vi "FL_Preprocess_and_save_incrementally_TDMS.vi"(0 "Temporary file output path":path, 1 "Loop iteration":i32, 2 "Offsets, swaps and rotations":T2, 3 "Loop speed in ms":u16, 4 "Save every N seconds":u32=15, 5 "error in (no error)":errorcluster, 6 "Filter type":u16(ring)=5 items=["None", "Kalman 0.50", "Kalman 0.30", "Kalman 0.12", "Savitzky-Golay 3/5", "Savitzky-Golay 3/11", "Savitzky-Golay 3/31"], 7 "Sensor read input":T5(array[cluster]), 8 "Input cluster of SG coefficients":T1, 9 "tdms file in":refnum<k34>, 10 "Pixels per mm":dbl, 11 "Data flow controls in":T4, 12 "Diagram at recording bounds":T3, 13 "Sensor board size":string="Small") -> (14 "Eff. save interval":sgl, 15 "Latest sensor output (decoded)":string[][](array[string]), 16 "Fire TTL":bool, 17 "TTL out N":u8, 18 "Current TTL status":u8, 19 "error out":errorcluster)   [LabVIEW 2018, in "Tracker.lvlib"]
uses:
  Tracker.lvlib
  Controls/CTL_Data_flow_control_cluster.ctl
  <vilib>/Utility/miscctls.llb/LVBoundsTypeDef.ctl
  SW_Globals.vi
  <vilib>/Utility/file.llb/Write Delimited Spreadsheet (string).vi
panel:
  out "Bytes return count":u32
  out "VISA error out":errorcluster
  out "Output to the external terminal":string
  in  "Max chunk size":i64=100000
  in  "Number of the file chunk":u32
  out "Chunk size (in bytes)":i64
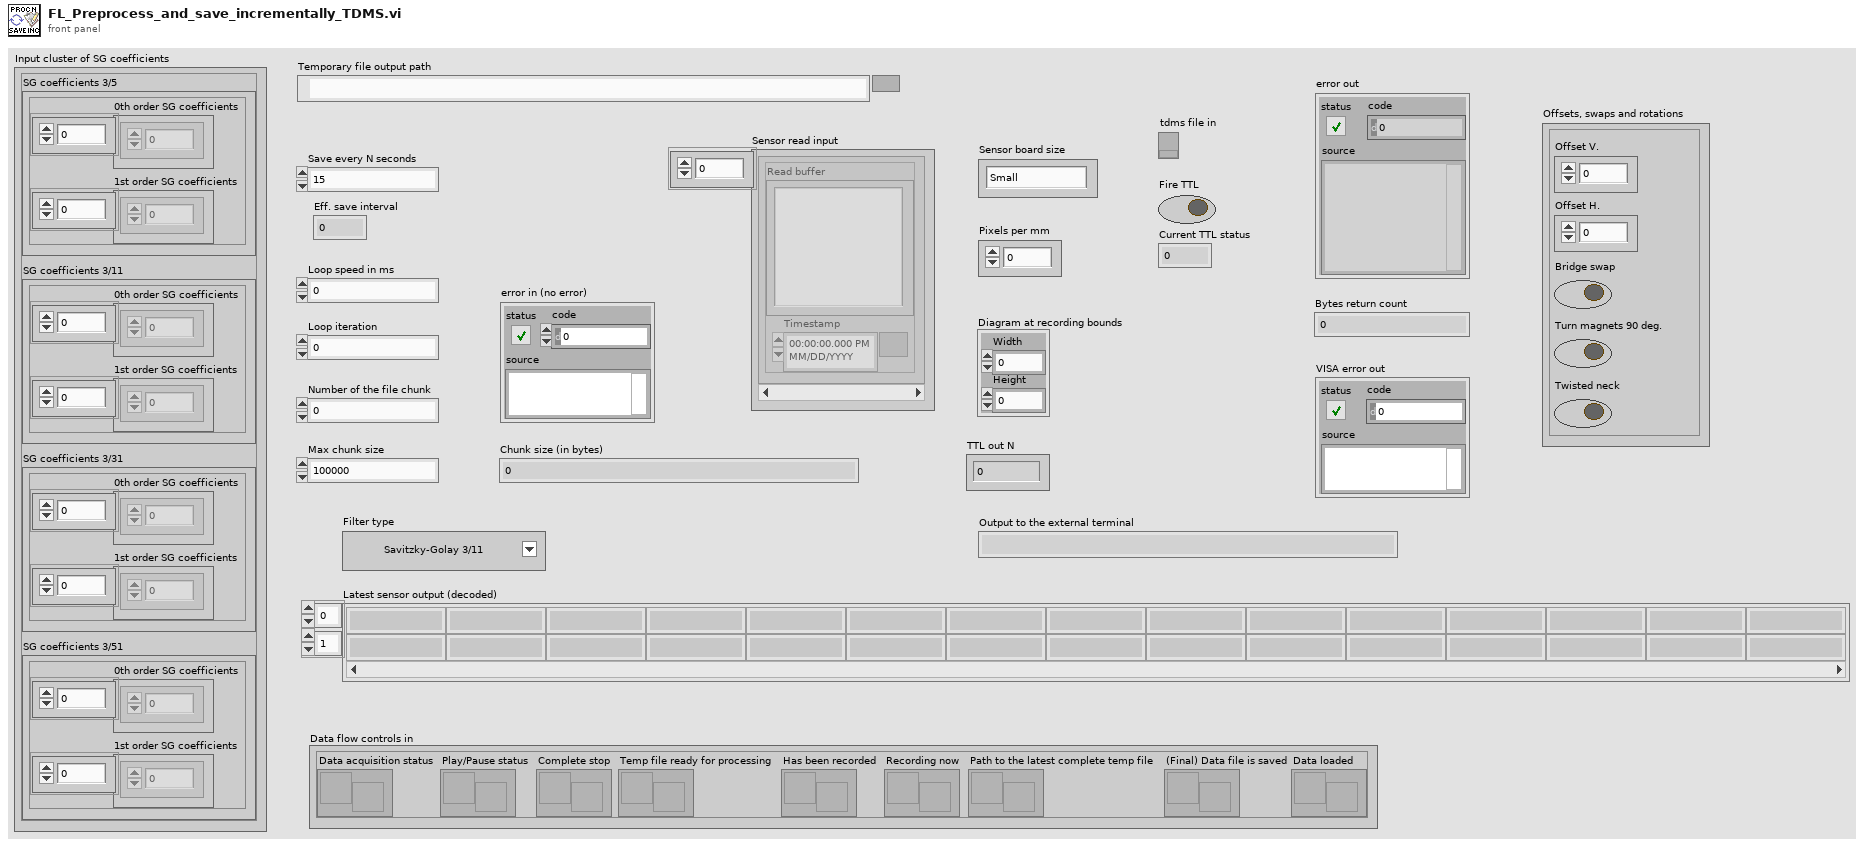
[diagram p1: front panel]
types:
  T1 = cluster{"SG coefficients 3/5":cluster{"0th order SG coefficients":dbl[], "1st order SG coefficients":dbl[]}, "SG coefficients 3/11":cluster{"0th order SG coefficients":dbl[], "1st order SG coefficients":dbl[]}, "SG coefficients 3/31":cluster{"0th order SG coefficients":dbl[], "1st order SG coefficients":dbl[]}, "SG coefficients 3/51":cluster{"0th order SG coefficients":dbl[], "1st order SG coefficients":dbl[]}}
  T2 = cluster{"Offset V.":sgl, "Offset H.":sgl, "Bridge swap":bool, "Turn magnets 90 deg.":bool, "Twisted neck":bool}
  T3 = typedef "LVBoundsTypeDef.ctl" = cluster{"Width":u32, "Height":u32}
  T4 = typedef "Tracker.lvlib/CTL_Data_flow_control_cluster.ctl" = cluster{"Data acquisition status":refnum<notifier>, "Play/Pause status":refnum<notifier>, "Complete stop":refnum<notifier>, "Temp file ready for processing":refnum<notifier>, "Has been recorded":refnum<notifier>, "Recording now":refnum<notifier>, "Path to the latest complete temp file":refnum<notifier>, "(Final) Data file is saved":refnum<notifier>, "Data loaded":refnum<notifier>}
  T5 = cluster{"Read buffer":string, "Timestamp":timestamp}[]
  T6 = cluster{"ms since ON":u32, "delta time":u32, "X1":sgl, "Y1":sgl, "X2":sgl, "Y2":sgl, "TTL inputs":u8, "TTL outputs":u8, "Frame timestamp":timestamp, "Frame OK":bool}
  T7 = cluster{"0th order SG coefficients":dbl[], "1st order SG coefficients":dbl[]}
  T8 = cluster{"X1 filtered":dbl, "Y1 filtered":dbl, "X2 filtered":dbl, "Y2 filtered":dbl, "X1 raw":dbl, "Y1 raw":dbl, "X2 raw":dbl, "Y2 raw":dbl}
  T9 = cluster{"R from center":dbl, "sin(a)":dbl, "Mouse Xc":dbl, "Mouse Yc":dbl, "X1-X2":dbl, "Y1-Y2":dbl, "Cage Xc":dbl, "Cage Yc":dbl}
  T10 = cluster{"R from center":dbl, "phi (mouse angular position in the cage)":dbl, "alpha (mouse rot. angle)":sgl, "X":dbl, "Y":dbl, "theta (from center towards mouse)":dbl, "beta (cage rot. against mouse)":sgl, "w (mouse angle to wall)":dbl}
  T11 = cluster{"Zone[1]":bool, "Zone[2]":bool, "Zone[3]":bool, "Zone[4]":bool, "Zone[5]":bool, "Zone[6]":bool, "Zone[7]":bool, "Zone[8]":bool, "Zone[9]":bool, "Zone[10]":bool, "Zone[11]":bool, "Zone[12]":bool, "Zone[13]":bool}
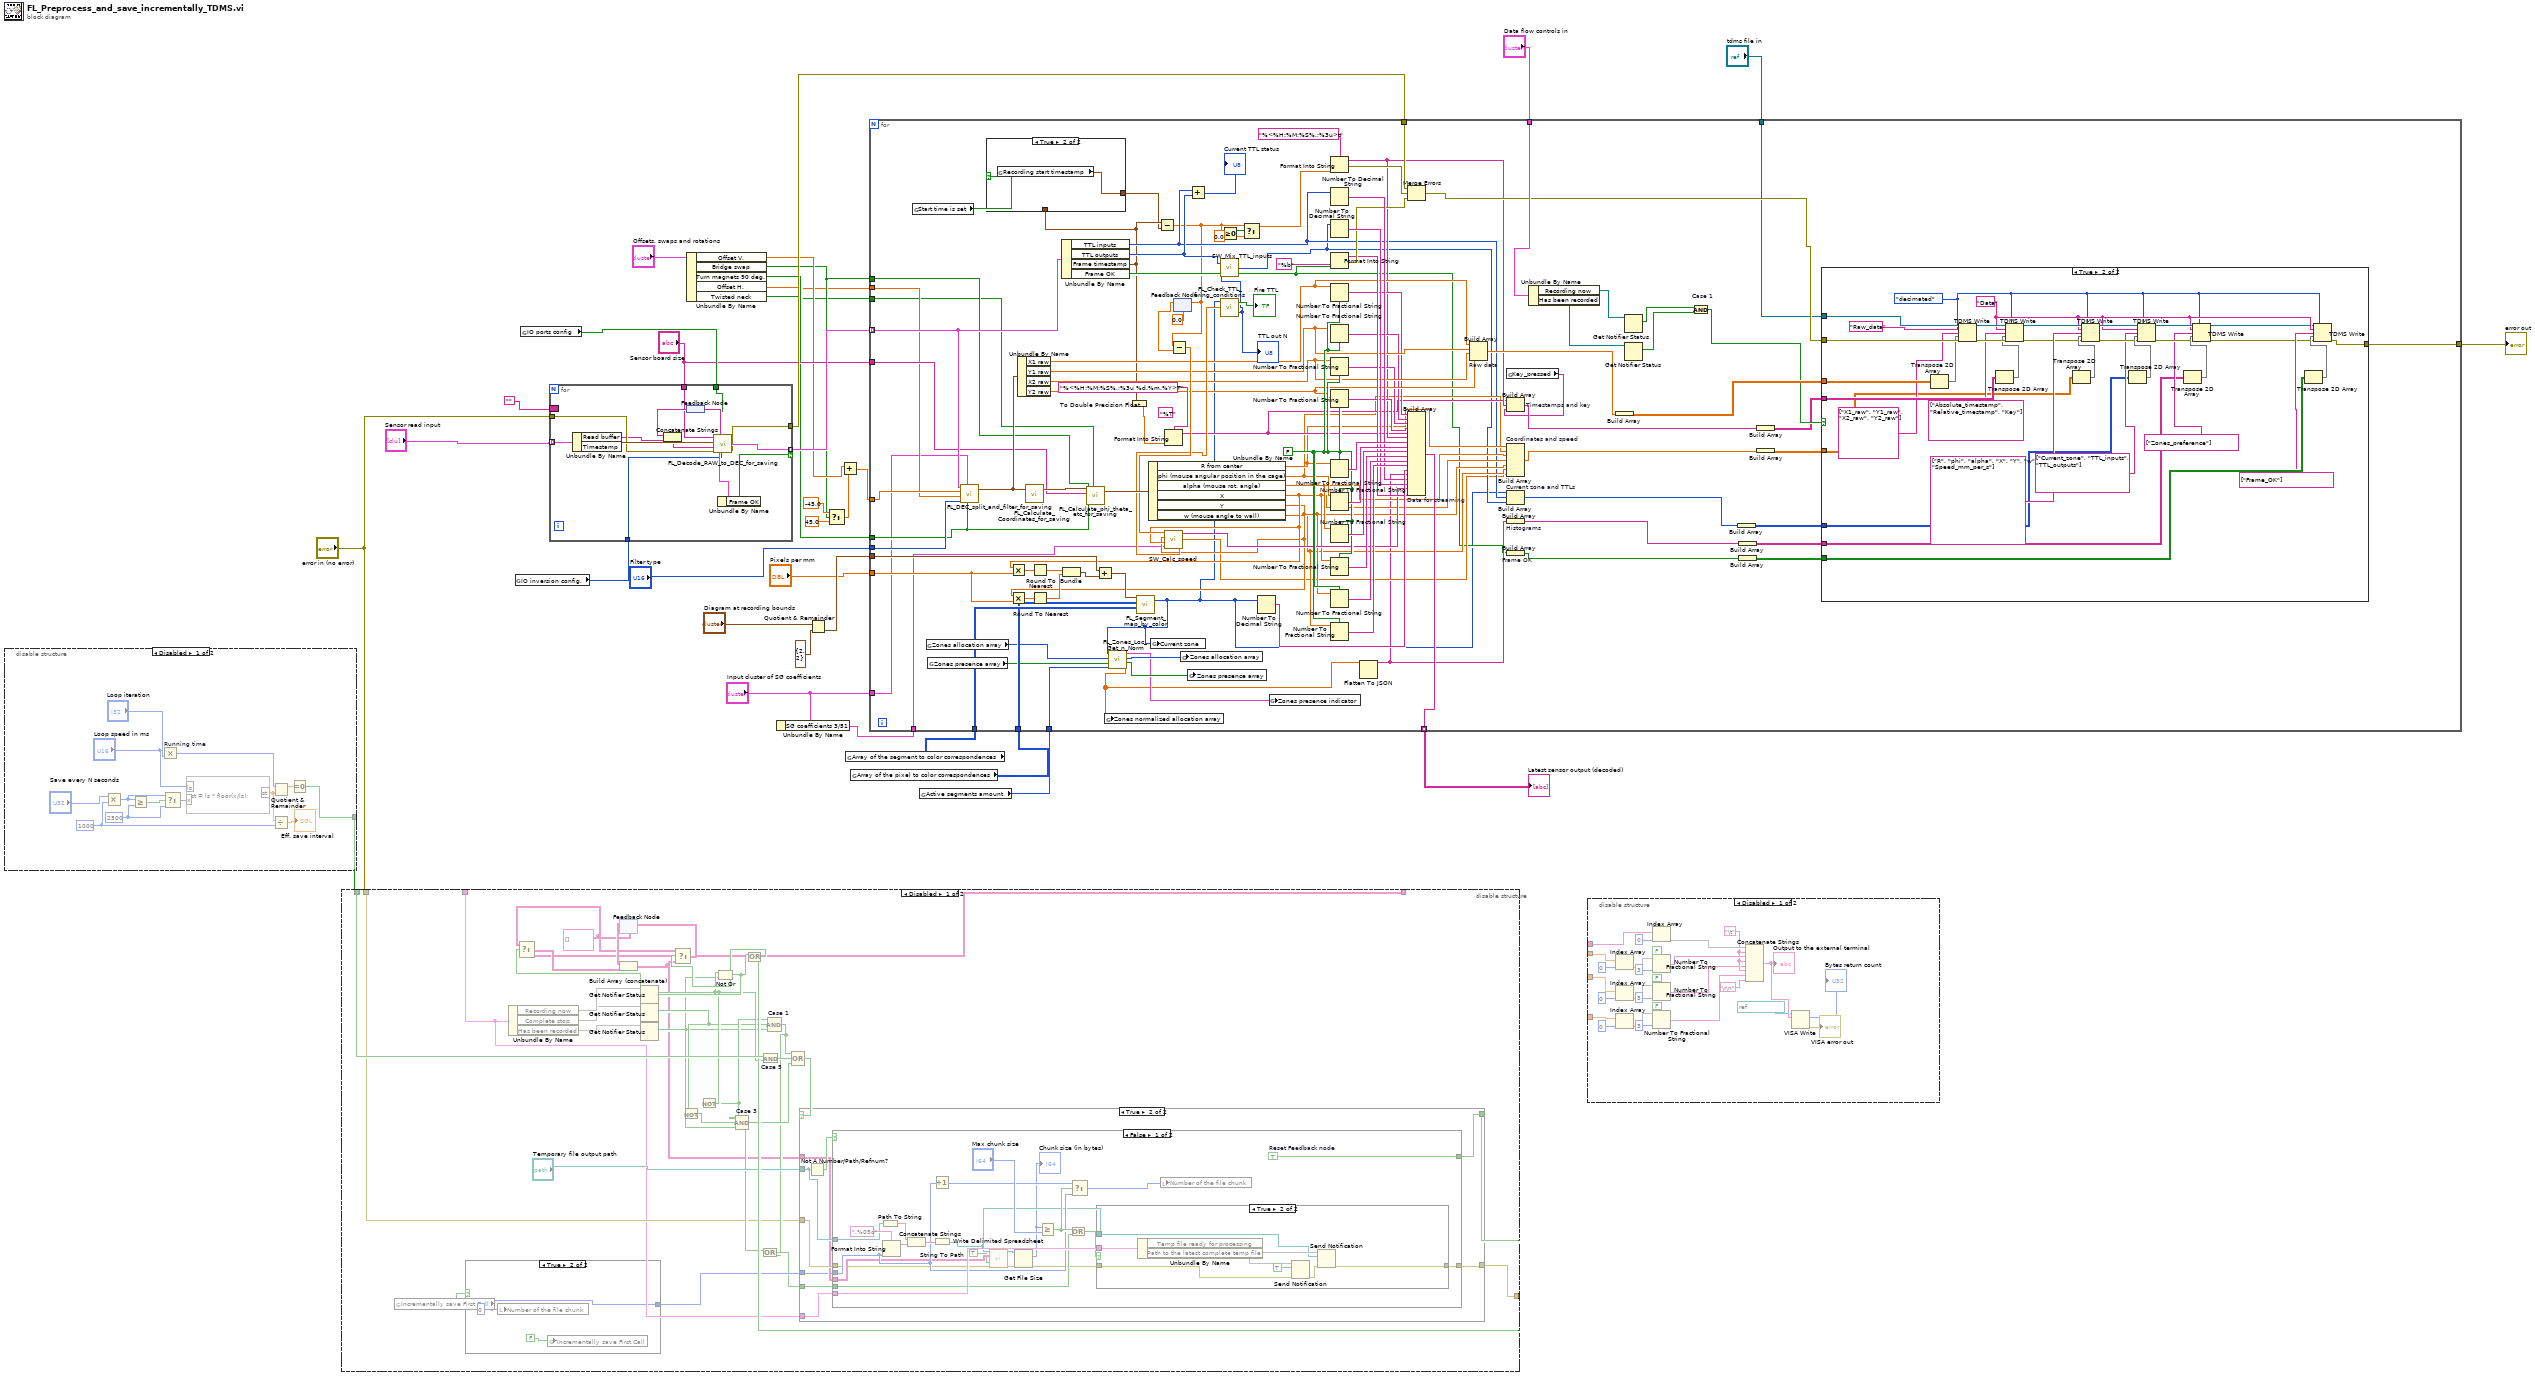
[diagram p0: block diagram]
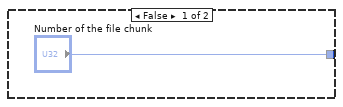
[diagram p2: hidden frame]
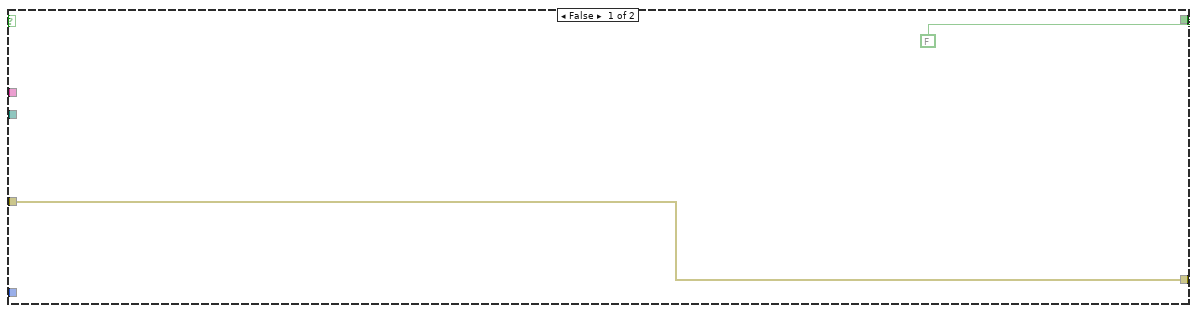
[diagram p3: hidden frame]
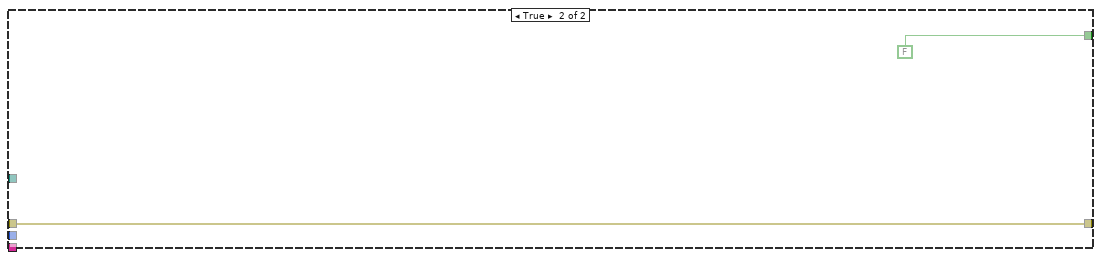
[diagram p5: hidden frame]
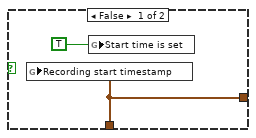
[diagram p9: hidden frame]
diagram:
  n1 = disable-structure shown="Disabled" {
    disable-tunnel: [w44 _] -> w33
    frame Disabled {
      w34 = u32 1000 ("y")
      w41 = 2500
      n2 = Multiply(x="Save every N seconds", y=w34) -> (x*y=w37:u32)
      n3 = Greater Or Equal?(x=w37, y=w41) -> (x >= y?=w42:bool)
      n4 = Multiply "Running time"(x="Loop speed in ms", y="Loop iteration") -> (x*y=w45:i32)
      n5 = Select(t=w37, s=w42, f=w41) -> (s? t:f=w39:u32)
      n6 = formula code="st = ls * floor(x/ls);"("ls"="Loop speed in ms", "x"=w39) -> ("st"=w36:dbl)
      n7 = Divide(x=w36, y=w34) -> (x/y=→"Eff. save interval":dbl)
      n8 = Quotient & Remainder(x=w45, y=w36) -> (x-y*floor(x/y)=w43:dbl)  [unwired: 1 out]
      n9 = Equal To 0?(x=w43) -> (x = 0?=w44:bool)
    }
    frame Enabled {
    }
  }
  n10 = disable-structure shown="Disabled" {
    disable-tunnel: w33 -> [w74 _]
    disable-tunnel: "error in (no error)" -> [w51 _]
    disable-tunnel: [w50 _] -> _
    disable-tunnel: _ -> [w48 _]
    disable-tunnel: _ -> [w47 _]
    frame Disabled {
      w62 = string[][] []
      n11 = global read "SW_Globals.vi" "Incrementally save First Call"() -> (w49:bool)
      n12 = case shown="True" w49 {
        tunnel: ["Number of the file chunk" w78] -> w65
        frame False {
        }
        frame True {
          w78 = 0 ("Number of the file chunk")
          n13 = local write "Number of the file chunk"(w78) -> ()
          n14 = global write "SW_Globals.vi" "Incrementally save First Call"(FALSE ("Incrementally save First Call")) -> ()
        }
      }
      n15 = Unbundle By Name(w47) -> ("Recording now"=w69, "Complete stop"=w68, "Has been recorded"=w67)
      n16 = feedback #1(w62) -> (w72:string[][])
      n17 = Get Notifier Status(notifier=w69) -> (current notification=w59:bool)  [unwired: 1 in, 4 out]
      n18 = Get Notifier Status(notifier=w68) -> (current notification=w57:bool)  [unwired: 1 in, 4 out]
      n19 = Get Notifier Status(notifier=w67) -> (current notification=w56:bool)  [unwired: 1 in, 4 out]
      n20 = Not(x=w57) -> (.not. x?=w55:bool)
      n21 = Not(x=w59) -> (.not. x?=w58:bool)
      n22 = Not Or(1:w56, 2:w59) -> (0:w61:bool)
      n23 = Select(t=w62, s=w61, f=w48) -> (s? t:f=w63:string[][])
      n24 = Build Array (concatenate)(w72, w63) -> (w52:string[][])
      n25 = Compound Arithmetic op=AND "Case 3"(w58, w55, w56) -> (w64:bool)
      n26 = And "Case 5"(x=w74, y=w59) -> (x .and. y?=w75:bool)
      n27 = Compound Arithmetic op=AND "Case 1"(w58, w57, w56) -> (w53:bool)
      n28 = Or(x=w64, y=w53) -> (x .or. y?=w54:bool)
      n29 = Compound Arithmetic op=OR(w53, w75, w64) -> (w73:bool)
      n30 = case shown="True" w73 {
        tunnel: "Temporary file output path" -> [_ w88]
        tunnel: [FALSE w87] -> w70
        tunnel: w51 -> [w79 w86]
        tunnel: [w79 w85] -> w50
        tunnel: w52 -> [_ w84]
        tunnel: w47 -> [_ w83]
        tunnel: w65 -> [_ w82]
        tunnel: w54 -> [_ w81]
        frame False {
        }
        frame True {
          n31 = Not A Number/Path/Refnum?(number/path/refnum=w88) -> (NaN/Path/Refnum?=w89:bool)
          n32 = case shown="False" w89 {
            tunnel: w88 -> [w104 _]
            tunnel: [w95 FALSE] -> w87
            tunnel: w86 -> [w91 w122]
            tunnel: [w102 w122] -> w85
            tunnel: w84 -> [w97 _]
            tunnel: w82 -> [w99 _]
            tunnel: w83 -> [w109 _]
            tunnel: w81 -> [w100 _]
            frame False {
              w95 = TRUE  # Reset Feedback node
              n33 = Path To String(path=w104) -> (string=w106:string)
              n34 = Format Into String(format string=".%05d", w99) -> (resulting string=w107:string)  [unwired: 2 in, 1 out]
              n35 = Concatenate Strings(w106, w107) -> (w108:string)
              n36 = Increment(x=w99) -> (x+1=w111:u32)
              n37 = String To Path(string=w108) -> (path=w98:path)
              n38 = call-poly <vilib>:"Write Delimited Spreadsheet.vi"("file path (dialog if empty)"=w98, "2D data"=w97, "append to file? (new file:F)"=TRUE, "error in (no error)"=w91) -> ("new file path (Not A Path if cancelled)"=w94:path, "error out"=w93:errorcluster)  [unwired: 10 in]
              n39 = Get File Size(file=w94, error in=w93) -> (size (in bytes)=w90:i64, 0:w92:errorcluster)  [unwired: 1 out]
              "Chunk size (in bytes)" <- w90
              n40 = Greater Or Equal?(x=w90, y="Max chunk size") -> (x >= y?=w103:bool)
              n41 = Or(x=w103, y=w100) -> (x .or. y?=w101:bool)
              n42 = Select(t=w111, s=w103, f=w99) -> (s? t:f=w110:u32)
              n43 = case shown="True" w101 {
                tunnel: w109 -> [_ w121]
                tunnel: w98 -> [_ w115]
                tunnel: w92 -> [w113 w117]
                tunnel: [w113 w116] -> w102
                frame False {
                }
                frame True {
                  n44 = Unbundle By Name(w121) -> ("Temp file ready for processing"=w120, "Path to the latest complete temp file"=w119)
                  n45 = Send Notification(notification=TRUE, notifier=w120, error in (no error)=w117) -> (error out=w118:errorcluster)  [unwired: 1 out]
                  n46 = Send Notification(notification=w115, notifier=w119, error in (no error)=w118) -> (error out=w116:errorcluster)  [unwired: 1 out]
                }
              }
              n47 = local write "Number of the file chunk"(w110) -> ()
            }
            frame True {
            }
          }
        }
      }
      n48 = Or(x=w61, y=w70) -> (x .or. y?=w60:bool)
      n49 = Select(t=w62, s=w60, f=w52) -> (s? t:f=w71:string[][])
      n50 = feedback-in #1(w71) -> ()
    }
    frame Enabled {
    }
  }
  n51 = global read "SW_Globals.vi" "IO inversion config."() -> (w16:u16)
  n52 = global read "SW_Globals.vi" "IO ports config"() -> (w18:bool[])
  n53 = for {
    tunnel: "Sensor read input" -> [w136] mode=indexing
    border: "" -> [_]
    tunnel: [w131] -> w30 mode=indexing if=w130
    tunnel: [w129] -> w31
    tunnel: "error in (no error)" -> [w128]
    tunnel: "Sensor board size" -> [w127]
    tunnel: w18 -> [w126]
    tunnel: w16 -> [w124]
    n54 = Unbundle By Name(w136) -> ("Read buffer"=w125:string, "Timestamp"=w135:timestamp)
    n55 = feedback #2() -> (w132:string)
    n56 = Concatenate Strings(w132, w125) -> (w134:string)
    n57 = call "FL_Decode_RAW_to_DEC_for_saving.vi"("Sensor board size"=w127, "IO ports config"=w126, "Input timestamp"=w135, "Input string"=w134, "IO inversion config."=w124, "Error In"=w128) -> ("Output string leftover"=w133:string, "DEC output cluster"=w131:T6, "Error Out"=w129:errorcluster)
    n58 = feedback-in #2(w133) -> ()
    n59 = Unbundle By Name(w131) -> ("Frame OK"=w130:bool)
  }
  n60 = Unbundle By Name("Offsets, swaps and rotations") -> ("Offset V."=w7:sgl, "Bridge swap"=w6:bool, "Turn magnets 90 deg."=w5:bool, "Offset H."=w4:sgl, "Twisted neck"=w3:bool)
  n61 = Unbundle By Name("Input cluster of SG coefficients") -> ("SG coefficients 3/51"=w1:T7)
  n62 = Quotient & Remainder(x="Diagram at recording bounds", y=T3 {"Width"=2, "Height"=2}) -> (floor(x/y)=w25:T3)  [unwired: 1 out]
  n63 = Select(t=sgl -45.0 ("x"), s=w6, f=sgl 45.0 ("x")) -> (s? t:f=w9:sgl)
  n64 = Add(x=w7, y=w9) -> (x+y=w19:sgl)
  n65 = global read "SW_Globals.vi" "Array of the segment to color correspondences"() -> (w23:u32[][])
  n66 = global read "SW_Globals.vi" "Array of the pixel to color correspondences"() -> (w22:u32[][])
  n67 = global read "SW_Globals.vi" "Active segments amount"() -> (w20:u8)
  n68 = for {
    tunnel: w30 -> [w243] mode=indexing
    tunnel: w31 -> [w231]
    tunnel: "Filter type" -> [w230]
    tunnel: w25 -> [w223]
    tunnel: "Pixels per mm" -> [w229]
    tunnel: w23 -> [w221]
    tunnel: w22 -> [w220]
    tunnel: w20 -> [w217]
    tunnel: w19 -> [w144]
    tunnel: w5 -> [w142]
    tunnel: "Sensor board size" -> [w199]
    tunnel: [w176] -> w15 mode=indexing
    tunnel: "tdms file in" -> [w188]
    tunnel: "Data flow controls in" -> [w191]
    tunnel: [w186] -> w12
    tunnel: w6 -> [w145]
    tunnel: w4 -> [w143]
    tunnel: w3 -> [w141]
    tunnel: "Input cluster of SG coefficients" -> [w140]
    tunnel: w1 -> [w139]
    w233 = FALSE ("use system decimal point (T)")
    (unwired) "%T" ("format string")
    n69 = global read "SW_Globals.vi" "Start time is set"() -> (w148:bool)
    n70 = global read "SW_Globals.vi" "Zones allocation array"() -> (w218:i32[])
    n71 = global read "SW_Globals.vi" "Zones presence array"() -> (w216:bool[])
    n72 = call "FL_DEC_split_and_filter_for_saving.vi"("Alternative magnets orientation"=w142, "Input cluster of SG coefficients"=w140, "Filter type"=w230, "Offset H."=w143, "Offset V."=w144, "DEC input cluster"=w243) -> ("Magnets coords"=w245:T8)  [unwired: 1 in]
    n73 = Unbundle By Name(w245) -> ("X1 raw"=w185:dbl, "Y1 raw"=w184:dbl, "X2 raw"=w183:dbl, "Y2 raw"=w182:dbl)
    n74 = call "FL_Calculate_Coordinates_for_saving.vi"("Magnets coords in"=w245) -> ("Output cluster of data"=w244:T9)  [unwired: 2 in]
    n75 = Unbundle By Name(w243) -> ("TTL inputs"=w167:u8, "TTL outputs"=w197:u8, "Frame timestamp"=w147:timestamp, "Frame OK"=w163:bool)
    n76 = case shown="True" w148 {
      tunnel: w147 -> [w246 _]
      tunnel: [w246 w248] -> w146
      frame False {
        n77 = global write "SW_Globals.vi" "Recording start timestamp"(w246) -> ()
        n78 = global write "SW_Globals.vi" "Start time is set"(TRUE ("Start time is set")) -> ()
      }
      frame True {
        n79 = global read "SW_Globals.vi" "Recording start timestamp"() -> (w248:timestamp)
      }
    }
    n80 = call "FL_Calculate_phi_theta_etc_for_saving.vi"("Input cluster of data"=w244, "Sensor board size"=w199, "Bridge swap"=w145, "Use alternative magnets orientation"=w142, "Clamp swap"=w141) -> ("Output data cluster"=w240:T10)  [unwired: 1 in]
    n81 = To Double Precision Float(number=w147) -> (double precision float=w201:dbl)
    n82 = Unbundle By Name(w240) -> ("R from center"=w173:dbl, "phi (mouse angular position in the cage)"=w172:dbl, "alpha (mouse rot. angle)"=w171:sgl, "X"=w170:dbl, "Y"=w169:dbl, "w (mouse angle to wall)"=w168:dbl)
    n83 = Multiply(x=w170, y=w229) -> (x*y=w228:dbl)
    n84 = Multiply(x=w169, y=w229) -> (x*y=w227:dbl)
    n85 = Round To Nearest(number=w228) -> (nearest integer value=w226:dbl)
    n86 = Round To Nearest(number=w227) -> (nearest integer value=w225:dbl)
    n87 = Bundle(w226, w225) -> (w224:cluster{dbl, dbl})  [unwired: 1 in]
    n88 = Add(x=w223, y=w224) -> (x+y=w222:cluster{dbl, dbl})
    n89 = call "FL_Segment_map_by_color.vi"("Array of the segment to color correspondences"=w221, "Array of the pixel to color correspondences"=w220, "Mouse abs. coordinates, pix"=w222) -> ("Current segment' number"=w138:u32)  [unwired: 1 in, 1 out]
    n90 = call "FL_Zones_Loc_Get_n_Norm.vi"("Amount of active segments"=w217, "Zones presence array in"=w216, "Zones allocation array in"=w218, "Current segment' number"=w138) -> ("Zones normalized allocation array out"=w210:dbl[], "Zones presence array out"=w214:bool[], "Zones allocation array out"=w215:i32[], "Zones presence indicator cluster out"=w213:T11)  [unwired: 4 in]
    n91 = global write "SW_Globals.vi" "Zones normalized allocation array"(w210) -> ()
    n92 = global write "SW_Globals.vi" "Current zone"(w138) -> ()
    n93 = Subtract(x=w147, y=w146) -> (x-y=w150:dbl)
    n94 = Format Into String(format string="%<%H:%M:%S%,;%3u %d.%m.%Y>T", w201) -> (resulting string=w174:string)  [unwired: 2 in, 1 out]
    n95 = feedback-in #3(w150) -> ()
    n96 = feedback #3(0.0) -> (w205:dbl)
    n97 = Subtract(x=w150, y=w205) -> (x-y=w203:dbl)
    n98 = call "SW_Calc_speed.vi"("SG coefficients"=w139, "X coord, mm"=w170, "Y coord, mm"=w169, "Time per frame, s"=w203) -> ("Mouse speed for TTL detection, mm/s"=w198:dbl, "Mouse speed, mm/s"=w165:dbl, "Mouse speed for saving, mm/s"=w202:string)
    n99 = global write "SW_Globals.vi" "Zones allocation array"(w215) -> ()
    n100 = global write "SW_Globals.vi" "Zones presence array"(w214) -> ()
    n101 = Add(x=w167, y=w197) -> (x+y=→"Current TTL status":u8)
    n102 = call "FL_Check_TTL_firing_conditions.vi"("Current speed, mm/s"=w198, "Current segment' number (last value)"=w138) -> ("TTL out N"=w196:u8, "Fire TTL"=→"Fire TTL":bool)  [unwired: 1 in]
    "TTL out N" <- w196
    n103 = call "SW_Mix_TTL_inputs.vi"("TTL input 2"=w196, "TTL input 1"=w197) -> ("TTL mixed output"=w166:u8)
    n104 = Greater Or Equal To 0?(x=w150) -> (x >= 0?=w151:bool)
    n105 = Select(t=w150, s=w151, f=0.0) -> (s? t:f=w152:dbl)
    n106 = Number To Decimal String(number=w138) -> (decimal integer string=w219:string)  [unwired: 1 in]
    n107 = global write "SW_Globals.vi" "Zones presence indicator"(w213) -> ()
    n108 = Format Into String(format string="%<%H:%M:%S%.;%3u>t", w152) -> (resulting string=w175:string, error out=w232:errorcluster)  [unwired: 2 in]
    n109 = Number To Decimal String(number=w167) -> (decimal integer string=w211:string)  [unwired: 1 in]
    n110 = Number To Decimal String(number=w166) -> (decimal integer string=w212:string)  [unwired: 1 in]
    n111 = Format Into String(format string="%b", w163) -> (resulting string=w204:string, error out=w209:errorcluster)  [unwired: 2 in]
    n112 = Number To Fractional String(use system decimal point (T)=w233, number=w185) -> (F-format string=w177:string)  [unwired: 2 in]
    n113 = Number To Fractional String(use system decimal point (T)=w233, number=w184) -> (F-format string=w178:string)  [unwired: 2 in]
    n114 = Number To Fractional String(use system decimal point (T)=w233, number=w183) -> (F-format string=w179:string)  [unwired: 2 in]
    n115 = Number To Fractional String(use system decimal point (T)=w233, number=w182) -> (F-format string=w180:string)  [unwired: 2 in]
    n116 = Number To Fractional String(use system decimal point (T)=w233, number=w173) -> (F-format string=w239:string)  [unwired: 2 in]
    n117 = Number To Fractional String(use system decimal point (T)=w233, number=w172) -> (F-format string=w238:string)  [unwired: 2 in]
    n118 = Number To Fractional String(use system decimal point (T)=w233, number=w171) -> (F-format string=w237:string)  [unwired: 2 in]
    n119 = Number To Fractional String(use system decimal point (T)=w233, number=w170) -> (F-format string=w236:string)  [unwired: 2 in]
    n120 = Number To Fractional String(use system decimal point (T)=w233, number=w169) -> (F-format string=w235:string)  [unwired: 2 in]
    n121 = Number To Fractional String(use system decimal point (T)=w233, number=w168) -> (F-format string=w234:string)  [unwired: 2 in]
    n122 = Flatten To JSON(anything=w210) -> (JSON string=w164:string)  [unwired: 2 in, 1 out]
    n123 = Merge Errors(w231, w232, w209) -> (w190:errorcluster)
    n124 = Build Array "Data for streaming"(w177, w178, w179, w180, w174, w175, w239, w238, w237, w236, w235, w234, w219, w164, w211, w212, w202, w204) -> (w176:string[])
    n125 = Build Array "Raw data"(w185, w184, w183, w182) -> (w181:dbl[])
    n126 = global read "SW_Globals.vi" "Key_pressed"() -> (w137:string)
    n127 = Build Array "Timestamps and key"(w174, w175, w137) -> (w162:string[])
    n128 = Build Array "Coordinates and speed"(w173, w172, w171, w170, w169, w168, w165) -> (w160:dbl[])
    n129 = Build Array "Current zone and TTLs"(w138, w167, w166) -> (w158:u32[])
    n130 = Build Array "Histograms"(w164) -> (w156:string[])
    n131 = Build Array "Frame OK"(w163) -> (w154:bool[])
    n132 = Unbundle By Name(w191) -> ("Recording now"=w192:refnum<notifier>, "Has been recorded"=w193:refnum<notifier>)
    n133 = Build Array(w181) -> (w189:dbl[][])
    n134 = Get Notifier Status(notifier=w192) -> (current notification=w194:bool)  [unwired: 1 in, 4 out]
    n135 = Get Notifier Status(notifier=w193) -> (current notification=w195:bool)  [unwired: 1 in, 4 out]
    n136 = And "Case 1"(x=w194, y=w195) -> (x .and. y?=w187:bool)
    n137 = Build Array(w158) -> (w157:u32[][])
    n138 = Build Array(w156) -> (w155:string[][])
    n139 = Build Array(w154) -> (w153:bool[][])
    n140 = Build Array(w162) -> (w161:string[][])
    n141 = Build Array(w160) -> (w159:dbl[][])
    n142 = case shown="True" w187 {
      tunnel: w190 -> [w249 w283]
      tunnel: [w249 w254] -> w186
      tunnel: w189 -> [_ w282]
      tunnel: w161 -> [_ w281]
      tunnel: w188 -> [_ w280]
      tunnel: w159 -> [_ w270]
      tunnel: w157 -> [_ w263]
      tunnel: w155 -> [_ w258]
      tunnel: w153 -> [_ w256]
      frame False {
      }
      frame True {
        w253 = "Data" ("group name in (Untitled)")
        w252 = enum16{"decimated", "interleaved"}."decimated" ("data layout (0:decimated)")
        n143 = Transpose 2D Array(2D array=w282) -> (transposed array=w278:dbl[][])
        n144 = TDMS Write(0:w280, 1:w252, 5:"Raw_data" ("group name in (Untitled)"), 7:string[] ["X1_raw", "Y1_raw", "X2_raw", "Y2_raw"] ("Columns Names"), 9:w278, 11:w283) -> (4:w276:refnum<k34>, 15:w275:errorcluster)  [unwired: 2 out]
        n145 = Transpose 2D Array(2D array=w281) -> (transposed array=w273:string[][])
        n146 = TDMS Write(0:w276, 1:w252, 5:w253, 7:string[] ["Absolute_timestamp", "Relative_timestamp", "Key"] ("Columns Names"), 9:w273, 11:w275) -> (4:w269:refnum<k34>, 15:w268:errorcluster)  [unwired: 2 out]
        n147 = Transpose 2D Array(2D array=w270) -> (transposed array=w272:dbl[][])
        n148 = TDMS Write(0:w269, 1:w252, 5:w253, 7:string[] ["R", "phi", "alpha", "X", "Y", "w", "Speed_mm_per_s"] ("Columns Names"), 9:w272, 11:w268) -> (4:w266:refnum<k34>, 15:w265:errorcluster)  [unwired: 2 out]
        n149 = Transpose 2D Array(2D array=w263) -> (transposed array=w267:u32[][])
        n150 = TDMS Write(0:w266, 1:w252, 5:w253, 7:string[] ["Current_zone", "TTL_inputs", "TTL_outputs"] ("Columns Names"), 9:w267, 11:w265) -> (4:w260:refnum<k34>, 15:w261:errorcluster)  [unwired: 2 out]
        n151 = Transpose 2D Array(2D array=w258) -> (transposed array=w262:string[][])
        n152 = TDMS Write(0:w260, 1:w252, 5:w253, 7:string[] ["Zones_preference"] ("Columns Names"), 9:w262, 11:w261) -> (4:w250:refnum<k34>, 15:w251:errorcluster)  [unwired: 2 out]
        n153 = Transpose 2D Array(2D array=w256) -> (transposed array=w257:bool[][])
        n154 = TDMS Write(0:w250, 1:w252, 5:w253, 7:string[] ["Frame_OK"] ("Columns Names"), 9:w257, 11:w251) -> (15:w254:errorcluster)  [unwired: 3 out]
      }
    }
  }
  "Latest sensor output (decoded)" <- w15
  "error out" <- w12
  n155 = disable-structure shown="Disabled" {
    disable-tunnel: _ -> [w310 _]
    disable-tunnel: _ -> [w305 _]
    disable-tunnel: _ -> [w304 _]
    disable-tunnel: _ -> [w303 _]
    frame Disabled {
      w291 = "\t"
      n156 = Index Array(array=w305, index=0) -> (element=w302)
      n157 = Index Array(array=w304, index=0) -> (element=w297)
      n158 = Index Array(array=w303, index=0) -> (element=w294)
      n159 = Index Array(array=w310, index=0) -> (element=w293)
      n160 = Number To Fractional String(use system decimal point (T)=FALSE, number=w302, precision (6)=i16 3) -> (F-format string=w292:string)  [unwired: 1 in]
      n161 = Number To Fractional String(use system decimal point (T)=FALSE, number=w297, precision (6)=i16 3) -> (F-format string=w290:string)  [unwired: 1 in]
      n162 = Number To Fractional String(use system decimal point (T)=FALSE, number=w294, precision (6)=i16 3) -> (F-format string=w289:string)  [unwired: 1 in]
      n163 = Concatenate Strings(w293, w291, w292, w291, w290, w291, w289, "\r\n") -> (w287:string)
      "Output to the external terminal" <- w287
      n164 = VISA Write(VISA resource name=refnum<visa-resource-name> "COMTEST", write buffer=w287) -> (return count=→"Bytes return count":u32, error out=→"VISA error out":errorcluster)  [unwired: 1 in, 1 out]
    }
    frame Enabled {
    }
  }
